vi "AlliGator Build Dataset Information String.vi"() -> (3 "Dataset Information String":string)   [LabVIEW 2021, in "AlliGator Dataset Information Window.lvlib"]
doc: "Creates <B>Dataset Information String</B> based on internal variables and settings."
uses:
  AlliGator Dataset Information Window.lvlib
  AlliGator Variables List.ctl
  AlliGator Settings List.ctl
  Variant/Variant to Data/Variant to String.vi
  Variant/Variant to Data/Variant to I32.vi
  Variant/Variant to Data/Variant to Boolean.vi
  Variant/Variant to Data/Variant to Path.vi
  AlliGator Globals, Variables & Constants.lvlib
  Variant/Variant to Data/Variant to Data.lvlib
  AlliGator Settings.lvlib
  AlliGator Files.lvlib
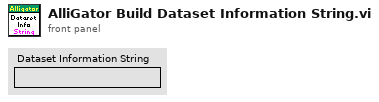
[diagram p1: front panel]
types:
  T1 = typedef "AlliGator Globals, Variables & Constants.lvlib/AlliGator Variables List.ctl" = enum16{"---- GUI ----", "Initialization Status", "State Indicators Refnum", "Original AlliGator Menu Items", "Current Action Loop State", "Script in progress", "Playback", "Loop Playback", "Search ROI Used", "Search ROI", "Decay Graph Max Legend Size", "Intensity Graph Max Legend Size", "Decay Statistics Graph Max Legend Size", "Phasor Graph Max Legend Size", "Phasor Ratio Graph Max Legend Size", "Lifetime Graph Max Legend Size", "---- Files ----", "Export Dataset Frames as Individual Files", "Show Batch Export Help Balloons", "Frames in Dataset", "ptu File Frame Start Indices", "Current Frame in Dataset", "Current Frame Timestamp", "------ Python Plugins ------", "Python Plugins Information", "Python Session", "Valid Python Session?", "---- Source Image ----", "Dataset Loaded", "Dataset Metadata", "Dataset Channel", "Dataset Data Description", "Background Dataset Metadata", "Background Dataset Channel", "Background Dataset Data Description", "Background File Subtraction", "Background File Path", "Background File Pile-up Correction", "Background File Pixel Well Capacity", "Background File Scaling Factor", "Source Image ROIs", "Current Source Image ROI", "Source Image ROI Event Refnum", "X_Source Image Display Range", "X_Source Image Palette Information", "Source Image Palette List", "Source Image Scale", "Current Dataset Load Settings", "Source Image:ROI Overlay Color", "---- Image Profile Window ----", "Image Profile:Overlay ROI in Source Image", "Image Profile Window Event Refnum", "Image Profile:IntensityType", "Image Profile:Intensity Average Type", "Image Profile:Intensity-weighted SDV", "Image Profile:Box Profile Type", "Image Profile Window Open", "Image Profile:Plotted Fit Parameter", "X_Type of Displayed Image", "X_Time Gate Slider", "Dataset Path", "Source Image Overlay to Erase", "Is Displayed Image Accumulated", "White Light Image Modified", "Mask Image Modified", "Macrotime Gate Separation", "------ Phasor Graph -------", "Phasor Graph:Show Line", "---- Phasor Plot ---", "Phasor Plot Parameters Changed", "FLI Dataset Modified since last Phasor Plot Calculation", "Phasor Harmonics Data", "Selected Phasor Harmonics", "Phasor Harmonic Manager Event Refnum", "Phasor Plot ROIs", "Current Phasor Plot ROI", "Phasor Plot ROI Event Refnum", "Phasor Plot Image Reference Points", "Phasor Plot Computed", "Phasor Plot Palette Information", "Phasor Plot Palette List", "Phasor Ratio Palette Information", "Phasor Ratio Palette List", "Phasor Image Scale", "Phasor Plot Image Overlay to Erase", "Phasor Plot Image Elements to Update", "Current Phasor Plot Calculation Parameters", "Current Phasor Calibration Options", "Reset Cumulated Phasor Plot", "Phasor Ratio Reference 1", "Phasor Ratio Lifetime Reference 1", "Phasor Ratio Reference 1 Frequency", "Phasor Ratio Reference 2", "Phasor Ratio Lifetime Reference 2", "Phasor Ratio Reference 2 Frequency", "---- Decay Analysis ----", "Number of Selected Decays to Fit", "LS Fit Results", "LAR Fit Results", "BS Fit Results", "Last Decay Max - Min", "Best Fit Parameters", "Best Fit Parameter Names", "Actual Size X", "Actual Size Y", "Binning X", "Binning Y", "Actual # Gates", "Dataset Number", "Gates to...", "Gates Skipped", "Gates to keep", "Gate Step", "Gate Separation", "Reversed Gates", "Pile-up Correction", "Pixel Well Capacity", "Background Subtracted", "Background Subtraction Method", "Background Definition Range", "Background File (deprecated)", "Number of Dataset Accumulated", "Array of Accumulated Dataset Paths", "Do Averaged Datasets", "Destination File Path", "Process Plot Target", "Use 1/D as Phasor Frequency", "---- Decay Fit Parameter Map -----", "Decay Fit Parameter Map Palette Information", "Decay Fit Parameter Map Palette List", "Local Decay Graph Window Event Refnum", "------- Local Decay Window ---------", "Use normalized IRF for convolution", "----- Miscellaneous ----", "Skippable Dialog Windows Status"}
  T2 = typedef "AlliGator Settings.lvlib/AlliGator Settings List.ctl" = enum16{"GUI:Visible Settings Tab", "GUI:Last Run Version", "Source Image:Use Image Histogram for Contrast", "Source Image:Low Count Pixels Rejection Options", "Source Image:High Count Pixels Rejection Options", "Source Image:Use Image Brightness", "Source Image:Blend Overlay with Image Background", "Source Image:Use Fixed ROI Diameter", "Source Image:ROI Diameter", "Source Image:ROI Center Color", "Source Image:Peak Threshold", "Source Image:Intensity Threshold", "Source Image:Image Binning Options", "Source Image:Image Smoothing Options", "Source Image:Image Histogram Active", "Source Image:Invert Binary Mask", "Source Image:Hot Pixel Removal", "Source Image:Overlay Analyzed ROI Center", "Source Image:Auto-Adjust Contrast", "Source Image:Histogram Lower Percentile", "Source Image:Histogram Upper Percentile", "Source Image:Save Source Image", "Source Image:Scale Bar Options", "Source Image:Image Resolution (Pixel Size)", "Data Information:Gate Width", "Data Information:Nanotime Gate Separation", "Data Information:Macrotime Gate Separation", "Data Information:Gate Step", "Data Information:# Gates", "Data Information:Gate Image Exposure", "Data Information:Gate Image Integration", "Data Information:Gates to Skip", "Data Information:Gates to Keep", "Data Information:Define Gates to", "Data Information:Channel Name", "Data Information:Available Channel Names", "Data Information:Channel Arithmetic", "Data Information:Background File Subtraction", "Data Information:Background File", "Data Information:Background Scaling Factor", "Data Information:Background Pile-up Correction", "Data Information:Background Pixel Well Capacity", "Data Information:Laser Period", "Data Information:SYNC Period", "Data Information:Pile-up Correction", "Data Information:Pixel Well Capacity", "Data Information:Dataset Scaling Factor", "Fluorescence Decay_Decay Pre-Processing:Reverse Gates", "Fluorescence Decay_Decay Pre-Processing:Verbose Decay Pre-Processing", "Fluorescence Decay_Decay Pre-Processing:Use Decay Pre-Processing", "Fluorescence Decay_Decay Pre-Processing:Background Subtraction", "Fluorescence Decay_Decay Pre-Processing:Background Definition Range", "Fluorescence Decay_Decay Pre-Processing:Baseline Subtraction Method", "Fluorescence Decay_Decay Pre-Processing:Operations Order", "Fluorescence Decay_Decay Pre-Processing:Smoothing Parameter", "Fluorescence Decay_Decay Pre-Processing:Shift Decay", "Fluorescence Decay_Decay Pre-Processing:Decay Shift Parameters", "Fluorescence Decay_Decay Pre-Processing:Fold Decay", "Fluorescence Decay_Decay Pre-Processing:# Folds", "Fluorescence Decay_Decay Pre-Processing:1-Normalize Decay", "Fluorescence Decay_Decay Pre-Processing:[0-1]-Normalize Decay", "Fluorescence Decay_Decay Pre-Processing:Smoothen Decay", "Fluorescence Decay_Decay Pre-Processing:Extrapolate Decay", "Fluorescence Decay_Decay Pre-Processing:Use Periodicity", "Fluorescence Decay_Decay Pre-Processing:Use Cursors", "Fluorescence Decay_Decay Pre-Processing:Tail Fraction", "Fluorescence Decay_Decay Pre-Processing:Head Fraction", "Fluorescence Decay_Decay Pre-Processing:Additional Points", "Fluorescence Decay_Decay Pre-Processing:Straighten Decay", "Fluorescence Decay_Decay Pre-Processing:Constant Background", "Fluorescence Decay_Decay Pre-Processing:Pixel-Normalize Decay", "Fluorescence Decay_Advanced Analysis:Extract IRF instead of Decay", "Fluorescence Decay_Advanced Analysis:IRF Extraction Options", "Fluorescence Decay_Advanced Analysis:IRF Optimization Options", "Fluorescence Decay_Advanced Analysis:Square Pulse Options", "Fluorescence Decay_Advanced Analysis:IRF Order", "Fluorescence Decay_Advanced Analysis:IRF Time Constants", "Fluorescence Decay_Advanced Analysis:Wavelet Analysis Options", "Fluorescence Decay_Advanced Analysis:Average Lifetime Options", "Fluorescence Decay_Fit Options:Fit Options", "Fluorescence Decay_Fit Options:Use Legacy Fitting Approach", "Fluorescence Decay_Fit Options:Use Data Information Laser Period", "Fluorescence Decay_Fit Parameters:Displayed Fit Parameters", "Fluorescence Decay_Fit Parameters:Fit Parameter Constraints", "Fluorescence Decay_Fit Parameters:Export Tabulated Results", "Fluorescence Decay_Fit Parameters:MLE Baseline Offset Type", "Fluorescence Decay_Fit Parameters:MLE Baseline Offset", "Fluorescence Decay_Fit Parameters:Guess Parameter Names", "Fluorescence Decay_Fit Parameters:Guess Parameter Values", "Fluorescence Decay_Fit Parameters:Guess Parameters Options", "Fluorescence Decay_Styles:Show Last Decay Only", "Fluorescence Decay_Styles:Decay Graph Color Array", "Fluorescence Decay:Decay Graph Active", "Fluorescence Decay Statistics:Min Peak Value", "Fluorescence Decay Statistics:Reject Low Decay Peak Pixels", "Fluorescence Decay Statistics:Reject High Decay Peak Pixels", "Fluorescence Decay Statistics:Max Peak Value", "Time Traces:Use File Timestamp", "Time Traces:Time Step", "Time Traces:Use Intensity Correction File", "Time Traces:Intensity Correction File", "Phasor Plot:Phasor Plot Smoothing Options", "Phasor Plot:Phasor Plot Size", "Phasor Plot:Phasor Plot Graphics Options", "Phasor Plot:Cumulative Phasor Plot", "Phasor Plot:Use Phasor Brightness", "Phasor Plot:Blend Overlay with Phasor Background", "Phasor Plot:Save Phasor Plot", "Phasor Plot:Show References", "Phasor Plot:Phasor Ratio Decay Range", "Phasor Plot:Exponential Fading", "Phasor Plot:Phasor Ratio Reference Colors", "Phasor Plot:Reference Radius", "Phasor Plot:Show Color Map Vertices", "Phasor Plot:Phasor Plot Active", "Phasor Plot:Phasor Ratio Color Map Type", "Phasor Plot:Phasor Ratio Color Map", "Phasor Plot:Phasor Ratio Display Range", "Phasor Plot:Selected Image ROI(s)", "Phasor Plot:All Image ROIs", "Phasor Plot:Selected Phasor Plot ROI(s)", "Phasor Plot:All Phasor Plot ROIs", "Phasor Plot:Phasor Ratio Color-Coded Quantity", "Phasor Plot:Store Phasor Harmonics", "Phasor Plot:Draw Reference Segment", "Phasor Plot:User-Defined Quantity", "Phasor Graph:Phasor Frequency", "Phasor Graph:Phasor Ratio Type", "Phasor Graph:Pixel-level Phasor Computation", "Phasor Graph:Save Phasor Graph", "Phasor Graph:Phasor Graph Active", "Phasor Graph:Phasor SDV Options", "Phasor Calibration:Use Backup Calibration if needed", "Phasor Graph:Define Shortest Lifetime as", "Phasor Calibration:Backup Calibration Type", "Phasor Calibration:Calibration Type", "Phasor Calibration:Calibration Lifetime", "Phasor Calibration:Calibration Map Algorithm", "Single-Exponential Phasor Locus (SEPL):Gate Parameters", "Single-Exponential Phasor Locus (SEPL):User-defined Gate", "Single-Exponential Phasor Locus (SEPL):User-defined IRF", "Single-Exponential Phasor Locus (SEPL):Phasor Parameters", "Single-Exponential Phasor Locus (SEPL):Decay & IRF Parameters", "Single-Exponential Phasor Locus (SEPL):Display Parameters", "Lifetime Analysis:Decay Analysis Parameters", "Lifetime Analysis:Lifetime Map Active", "Plugins:Python Settings", "Miscellaneous:Verbose Mode", "Miscellaneous:Beep after Script", "Miscellaneous:Saved Image File Format", "Miscellaneous:Exported Gate Image Settings", "Miscellaneous:Include Loading in Timing", "Miscellaneous:Verbose Settings Mode", "Miscellaneous:Histogram Options", "Miscellaneous:Beep on Error", "Miscellaneous:# Logical Processors Used", "Miscellaneous:ROI Description Max Characters", "Miscellaneous:Verbose Error Mode", "Miscellaneous:Transparent Mask Color"}
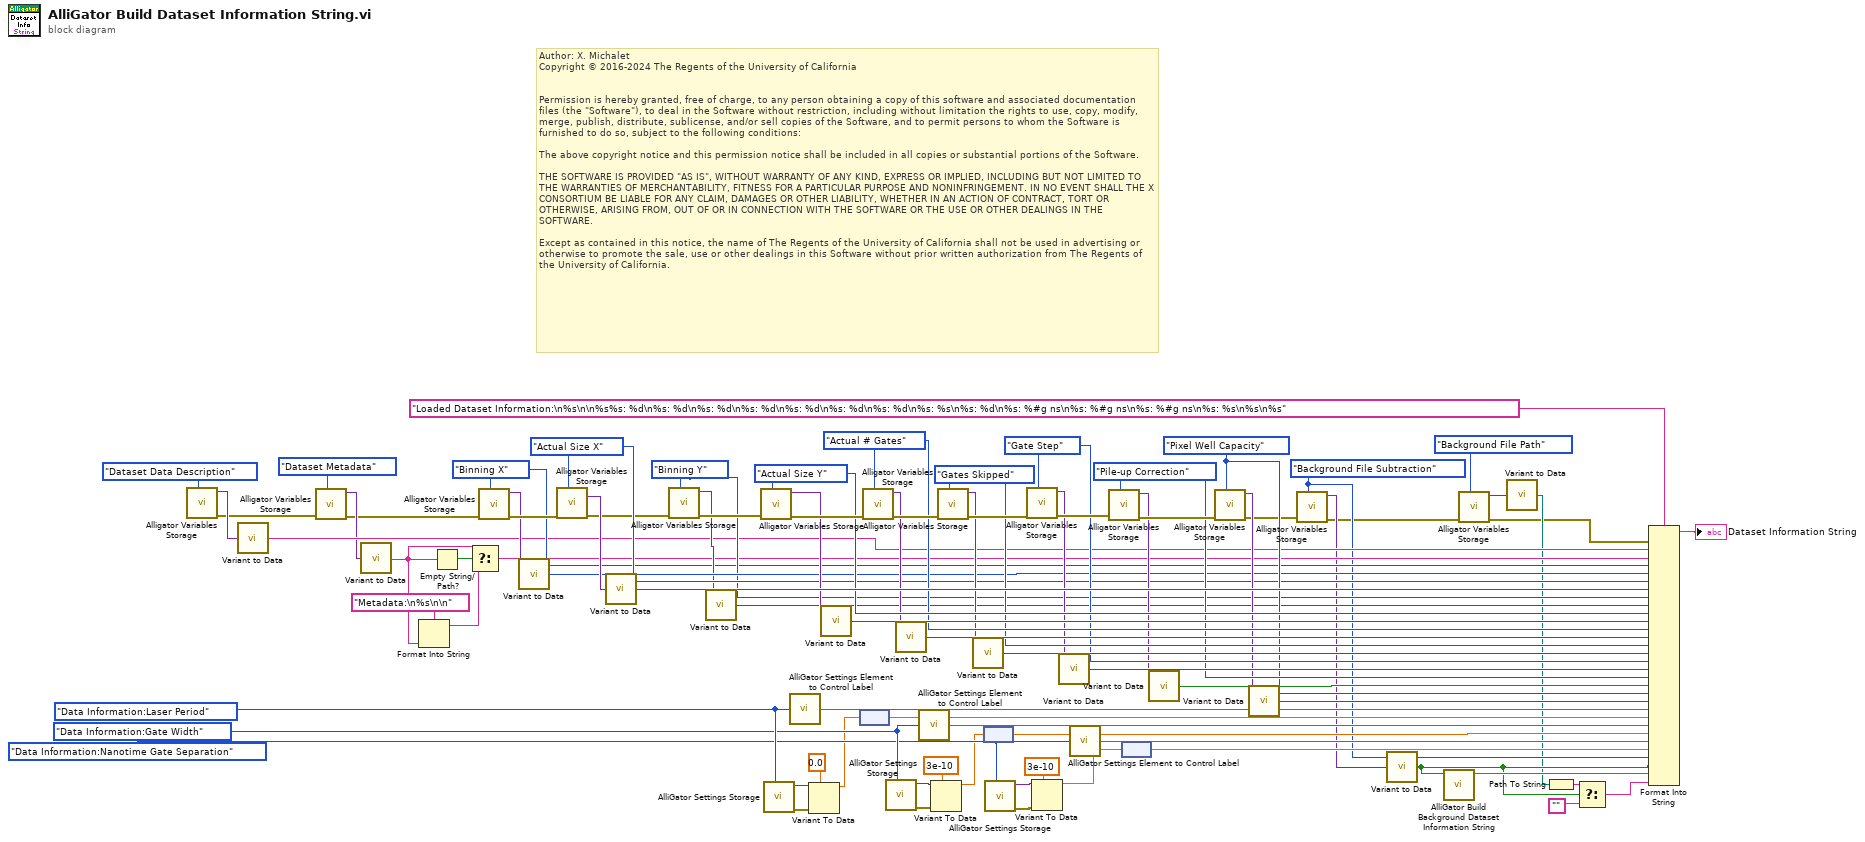
[diagram p0: block diagram]
diagram:
  w12 = AlliGator_Variables_List."Background File Subtraction" ("Alligator Variable")
  w27 = AlliGator_Variables_List."Binning Y" ("Alligator Variable")
  w24 = AlliGator_Variables_List."Binning X" ("Alligator Variable")
  w46 = AlliGator_Settings_List."Data Information:Gate Width" ("AlliGator Settings List")
  w47 = AlliGator_Settings_List."Data Information:Laser Period" ("AlliGator Settings List")
  w45 = AlliGator_Settings_List."Data Information:Nanotime Gate Separation" ("AlliGator Settings List")
  w63 = AlliGator_Variables_List."Gate Step" ("Alligator Variable")
  w66 = AlliGator_Variables_List."Gates Skipped" ("Alligator Variable")
  w57 = AlliGator_Variables_List."Pixel Well Capacity" ("Alligator Variable")
  w60 = AlliGator_Variables_List."Pile-up Correction" ("Alligator Variable")
  w69 = AlliGator_Variables_List."Actual # Gates" ("Alligator Variable")
  w72 = AlliGator_Variables_List."Actual Size Y" ("Alligator Variable")
  w32 = AlliGator_Variables_List."Actual Size X" ("Alligator Variable")
  # "Author: X. Michalet\nCopyright © 2016-2024 The Regents of the University of California\n \n\nPermission is hereby granted, free of charge, to any person obtaining a copy of this software and associated documentation files (the \"Software\"), to deal in the Software without restriction, including without limitation the rights to use, copy, modify, merge, publish, distribute, sublicense, and/or sell copies of the Software, and to permit persons to whom the Software is furnished to do so, subject to the following conditions:\n\nThe above copyright notice and this permission notice shall be included in all copies or substantial portions of the Software.\n\nTHE SOFTWARE IS PROVIDED \"AS IS\", WITHOUT WARRANTY OF ANY KIND, EXPRESS OR IMPLIED, INCLUDING BUT NOT LIMITED TO THE WARRANTIES OF MERCHANTABILITY, FITNESS FOR A PARTICULAR PURPOSE AND NONINFRINGEMENT. IN NO EVENT SHALL THE X CONSORTIUM BE LIABLE FOR ANY CLAIM, DAMAGES OR OTHER LIABILITY, WHETHER IN AN ACTION OF CONTRACT, TORT OR OTHERWISE, ARISING FROM, OUT OF OR IN CONNECTION WITH THE SOFTWARE OR THE USE OR OTHER DEALINGS IN THE SOFTWARE.\n\nExcept as contained in this notice, the name of The Regents of the University of California shall not be used in advertising or otherwise to promote the sale, use or other dealings in this Software without prior written authorization from The Regents of the University of California."
  n1 = call "Alligator Variables Storage.vi"("AlliGator Variable"=AlliGator_Variables_List."Dataset Data Description" ("Alligator Variable")) -> ("Error Out"=w20:errorcluster, "Data out"=w82:variant)  [unwired: 8 in, 1 out]
  n2 = call-poly "Variant to Data.vi"("Variant"=w82) -> ("String"=w23:string)  [unwired: 8 in]
  n3 = call "Alligator Variables Storage.vi"("AlliGator Variable"=AlliGator_Variables_List."Dataset Metadata" ("Alligator Variable"), "Error In"=w20) -> ("Error Out"=w19:errorcluster, "Data out"=w22:variant)  [unwired: 7 in, 1 out]
  n4 = call-poly "Variant to Data.vi"("Variant"=w22) -> ("String"=w15:string)  [unwired: 8 in]
  n5 = Format Into String(format string="Metadata:\n%s\n\n", w15) -> (resulting string=w16:string)  [unwired: 2 in, 1 out]
  n6 = Empty String/Path?(string/path=w15) -> (empty?=w18:bool)
  n7 = Select(t=w15, s=w18, f=w16) -> (s? t:f=w17:string)
  n8 = call "Alligator Variables Storage.vi"("AlliGator Variable"=w24, "Error In"=w19) -> ("Error Out"=w33:errorcluster, "Data out"=w31:variant)  [unwired: 7 in, 1 out]
  n9 = call-poly "Variant to Data.vi"("Variant"=w31) -> ("Value"=w30:i32)  [unwired: 8 in]
  n10 = call "Alligator Variables Storage.vi"("AlliGator Variable"=w32, "Error In"=w33) -> ("Error Out"=w29:errorcluster, "Data out"=w74:variant)  [unwired: 7 in, 1 out]
  n11 = call-poly "Variant to Data.vi"("Variant"=w74) -> ("Value"=w73:i32)  [unwired: 8 in]
  n12 = call "Alligator Variables Storage.vi"("AlliGator Variable"=w27, "Error In"=w29) -> ("Error Out"=w28:errorcluster, "Data out"=w26:variant)  [unwired: 7 in, 1 out]
  n13 = call-poly "Variant to Data.vi"("Variant"=w26) -> ("Value"=w25:i32)  [unwired: 8 in]
  n14 = call "Alligator Variables Storage.vi"("AlliGator Variable"=w72, "Error In"=w28) -> ("Error Out"=w76:errorcluster, "Data out"=w71:variant)  [unwired: 7 in, 1 out]
  n15 = call "AlliGator Settings Storage.vi"("AlliGator Settings List"=w47) -> ("Error Out"=w53:errorcluster, "Variant Data out"=w54:variant)  [unwired: 9 in]
  n16 = call "AlliGator Settings Element to Control Label.vi"("AlliGator Settings List"=w47) -> ("Label"=w43:string)  [unwired: 8 in]
  n17 = Variant To Data(error in=w53, type=dbl[unit] 0.0 ("Laser Period"), Variant=w54) -> (data=w42:dbl[unit])  [unwired: 1 out]
  n18 = call-poly "Variant to Data.vi"("Variant"=w71) -> ("Value"=w70:i32)  [unwired: 8 in]
  n19 = node(w42) -> (w41:dbl)
  n20 = call "Alligator Variables Storage.vi"("AlliGator Variable"=w69, "Error In"=w76) -> ("Error Out"=w78:errorcluster, "Data out"=w68:variant)  [unwired: 7 in, 1 out]
  n21 = call "AlliGator Settings Storage.vi"("AlliGator Settings List"=w46) -> ("Error Out"=w51:errorcluster, "Variant Data out"=w52:variant)  [unwired: 9 in]
  n22 = call-poly "Variant to Data.vi"("Variant"=w68) -> ("Value"=w67:i32)  [unwired: 8 in]
  n23 = call "AlliGator Settings Element to Control Label.vi"("AlliGator Settings List"=w46) -> ("Label"=w40:string)  [unwired: 8 in]
  n24 = Variant To Data(error in=w51, type=dbl[unit] 3e-10 ("Gate Duration"), Variant=w52) -> (data=w39:dbl[unit])  [unwired: 1 out]
  n25 = call "Alligator Variables Storage.vi"("AlliGator Variable"=w66, "Error In"=w78) -> ("Error Out"=w79:errorcluster, "Data out"=w65:variant)  [unwired: 7 in, 1 out]
  n26 = call-poly "Variant to Data.vi"("Variant"=w65) -> ("Value"=w64:i32)  [unwired: 8 in]
  n27 = node(w39) -> (w38:dbl)
  n28 = call "AlliGator Settings Storage.vi"("AlliGator Settings List"=w45) -> ("Error Out"=w49:errorcluster, "Variant Data out"=w50:variant)  [unwired: 9 in]
  n29 = call "Alligator Variables Storage.vi"("AlliGator Variable"=w63, "Error In"=w79) -> ("Error Out"=w80:errorcluster, "Data out"=w62:variant)  [unwired: 7 in, 1 out]
  n30 = Variant To Data(error in=w49, type=dbl[unit] 3e-10 ("Gate Duration"), Variant=w50) -> (data=w35:dbl[unit])  [unwired: 1 out]
  n31 = call-poly "Variant to Data.vi"("Variant"=w62) -> ("Value"=w61:i32)  [unwired: 8 in]
  n32 = call "AlliGator Settings Element to Control Label.vi"("AlliGator Settings List"=w45) -> ("Label"=w37:string)  [unwired: 8 in]
  n33 = call "Alligator Variables Storage.vi"("AlliGator Variable"=w60, "Error In"=w80) -> ("Error Out"=w77:errorcluster, "Data out"=w59:variant)  [unwired: 7 in, 1 out]
  n34 = node(w35) -> (w34:dbl)
  n35 = call-poly "Variant to Data.vi"("Variant"=w59) -> ("Value"=w58:bool)  [unwired: 8 in]
  n36 = call "Alligator Variables Storage.vi"("AlliGator Variable"=w57, "Error In"=w77) -> ("Error Out"=w13:errorcluster, "Data out"=w55:variant)  [unwired: 7 in, 1 out]
  n37 = call-poly "Variant to Data.vi"("Variant"=w55) -> ("Value"=w56:i32)  [unwired: 8 in]
  n38 = call "Alligator Variables Storage.vi"("AlliGator Variable"=w12, "Error In"=w13) -> ("Error Out"=w9:errorcluster, "Data out"=w11:variant)  [unwired: 7 in, 1 out]
  n39 = call-poly "Variant to Data.vi"("Variant"=w11) -> ("Value"=w6:bool)  [unwired: 8 in]
  n40 = call "AlliGator Build Background Dataset Information String.vi"("Bkgd Subtraction"=w6) -> ("Background Dataset Description"=w10:string)  [unwired: 9 in, 1 out]
  n41 = call "Alligator Variables Storage.vi"("AlliGator Variable"=AlliGator_Variables_List."Background File Path" ("Alligator Variable"), "Error In"=w9) -> ("Error Out"=w1:errorcluster, "Data out"=w7:variant)  [unwired: 7 in, 1 out]
  n42 = call-poly "Variant to Data.vi"("Variant"=w7) -> ("Path"=w5:path)  [unwired: 8 in]
  n43 = Path To String(path=w5) -> (string=w3:string)
  n44 = Select(t=w3, s=w6, f="") -> (s? t:f=w4:string)
  n45 = Format Into String(format string="Loaded Dataset Information:\n%s\n\n%s%s: %d\n%s: %d\n%s: %d\n%s: %d\n%s: %d\n%s: %d\n%s: %d\n%s: %s\n%s: %d\n%s: %#g ns\n%s: %#g ns\n%s: %#g ns\n%s: %s\n%s\n%s", error in=w1, w23, w17, w24, w30, w32, w73, w27, w25, w72, w70, w69, w67, w66, w64, w63, w61, w60, w58, w57, w56, w43, w41, w40, w38, w37, w34, w12, w6, w10, w4) -> (resulting string=→"Dataset Information String":string)  [unwired: 1 in, 1 out]
